vi "sample method.vi"(6 "Sample Commands":T2=enum."Index", 8 "error in (no error)":errorcluster, 9 "total run time":dbl[unit] format="%<%H:%M:%S%0u>t", 10 "current time":dbl[unit] format="%<%H:%M:%S>t", 11 "Ref cluster":T1) -> (0 "error out":errorcluster)   [LabVIEW 2012]
uses:
  Sample commands.ctl
  sample references.ctl
panel:
  in  "right white space":dbl=10.0
  in  "left white space":dbl=40.0
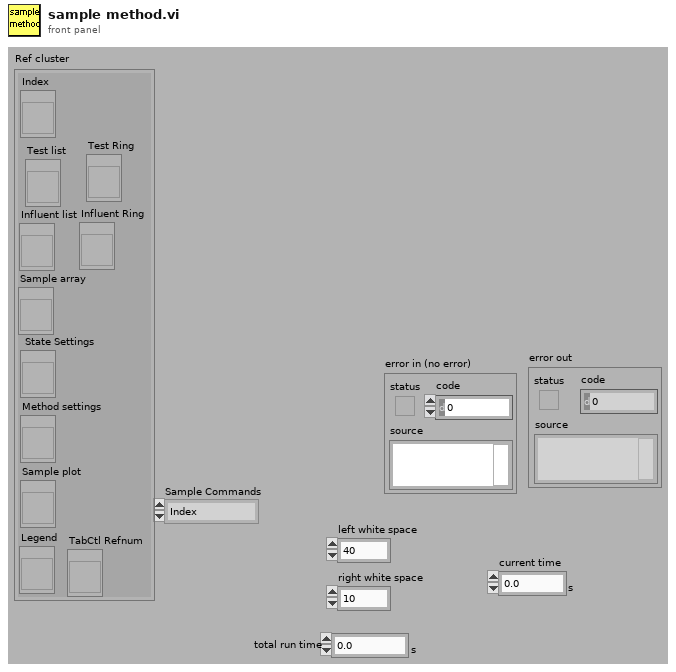
[diagram p1: front panel]
types:
  T1 = typedef "sample references.ctl" = cluster{"Index":refnum<vi>, "Test list":refnum<vi>, "Influent list":refnum<vi>, " State Settings":refnum<vi>, "Method settings":refnum<vi>, "Sample plot":refnum<vi>, "Legend":refnum<vi>, "Test Ring":refnum<vi>, "Influent Ring":refnum<vi>, "TabCtl Refnum":refnum<vi>, "Sample array":refnum<vi>}
  T2 = typedef "Sample commands.ctl" = enum16{"Configure", "Update times", "Index", "Update rings", "Plot current time"}
  T3 = cluster{"Width":u16, "Style":enum32{"Solid", "Dash", "Dot", "DashDot", "DashDotDot"}}
  T4 = typedef "Samples.ctl" = cluster{"start time":dbl[unit], "end time":dbl[unit], "state":string, "cycle":u16, "state":u16}[]
  T5 = cluster{"start time":dbl[unit], "end time":dbl[unit], "t/theta":dbl, "Test list":u16, "Influent list":u16, "Sample volume":dbl[unit], "Too close to previous sample":bool}[]
  T6 = typedef "LVBoundsTypeDef.ctl" = cluster{"Width":u32, "Height":u32}
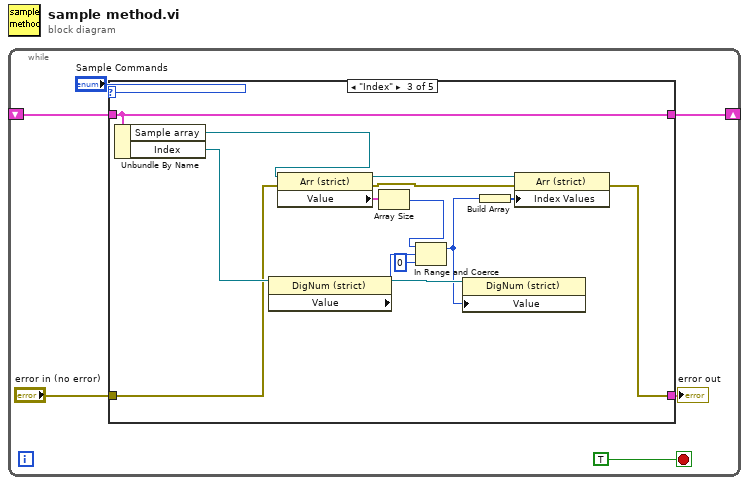
[diagram p0: block diagram]
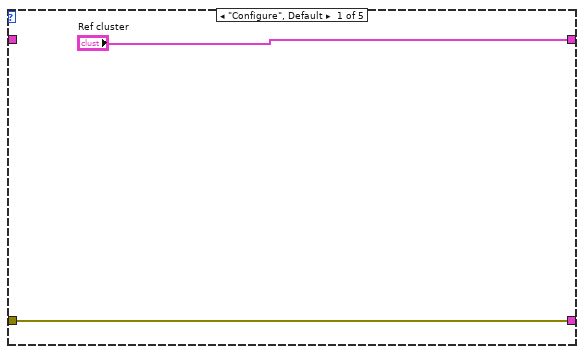
[diagram p2: hidden frame]
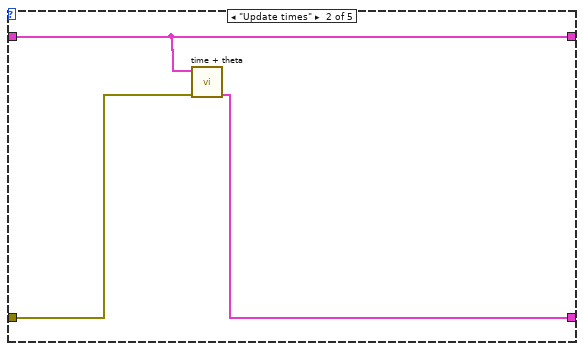
[diagram p3: hidden frame]
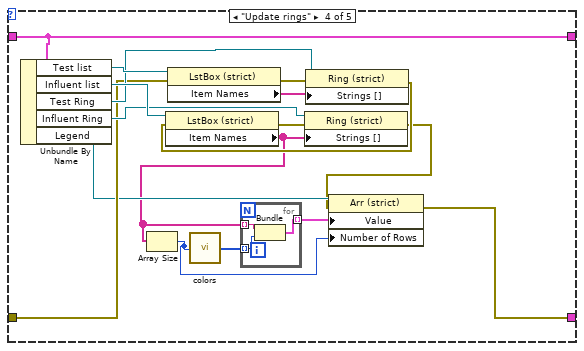
[diagram p4: hidden frame]
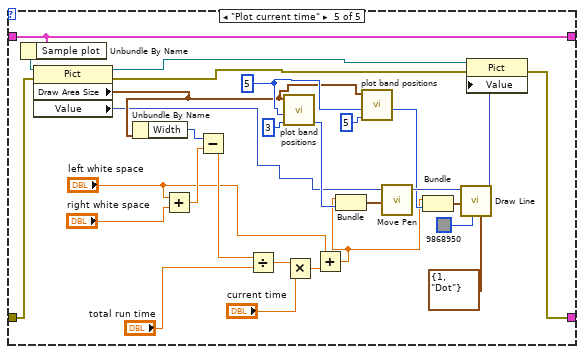
[diagram p5: hidden frame]
diagram:
  n1 = while {
    shift-right: [w4] -> _
    shift-left: _ -> [w3]
    stop <- TRUE stop-if-true
    n2 = case shown="\"Index\"" "Sample Commands" {
      tunnel: ["Ref cluster" w11 w15 w42 w54] -> w4
      tunnel: w3 -> [_ w11 w15 w42 w54]
      tunnel: "error in (no error)" -> [w8 w10 w14 w37 w48]
      tunnel: [w8 w9 w12 w27 w47] -> w1
      frame "Configure", Default {
      }
      frame "Update times" {
        n3 = call "time + theta.vi"("Sample start times"=w10, "Method settings"=w11) -> ("Samples"=w9:T4)  [unwired: 7 in, 2 out]
      }
      frame "Index" {
        n4 = Unbundle By Name(w15) -> ("Sample array"=w17:refnum<vi>, "Index"=w16:refnum<vi>)
        n5 = property class="DigNum (strict)"(reference=w16) -> (reference out=w20:refnum<vi>, "Value"=w21:i32)  [unwired: 1 in, 1 out]
        n6 = property class="Arr (strict)"(reference=w17, error in=w14) -> (reference out=w24:refnum<vi>, error out=w13:errorcluster, "Value"=w23:T5)
        n7 = Array Size(array=w23) -> (size(s)=w18:i32)
        n8 = In Range and Coerce(upper limit=w18, x=w21, lower limit=0) -> (coerced(x)=w19:i32)  [unwired: 1 out]
        n9 = property class="DigNum (strict)"(reference=w20, "Value"=w19) -> ()  [unwired: 1 in, 2 out]
        n10 = Build Array(w19) -> (w25:i32[])
        n11 = property class="Arr (strict)"(reference=w24, error in=w13, "Index Values"=w25) -> (error out=w12:errorcluster)  [unwired: 1 out]
      }
      frame "Update rings" {
        n12 = Unbundle By Name(w42) -> ("Test list"=w41:refnum<vi>, "Influent list"=w40:refnum<vi>, "Test Ring"=w39:refnum<vi>, "Influent Ring"=w38:refnum<vi>, "Legend"=w31:refnum<vi>)
        n13 = property class="LstBox (strict)"(reference=w41, error in=w37) -> (error out=w36:errorcluster, "Item Names"=w33:string[])  [unwired: 1 out]
        n14 = property class="Ring (strict)"(reference=w39, error in=w36, "Strings []"=w33) -> (error out=w35:errorcluster)  [unwired: 1 out]
        n15 = property class="LstBox (strict)"(reference=w40, error in=w35) -> (error out=w34:errorcluster, "Item Names"=w26:string[])  [unwired: 1 out]
        n16 = Array Size(array=w26) -> (size(s)=w30:i32)
        n17 = call "colors.vi"("colors needed"=w30) -> ("colors"=w32:u32[])
        n18 = for {
          tunnel: w26 -> [w45] mode=indexing
          tunnel: w32 -> [w44] mode=indexing
          tunnel: [w43] -> w29 mode=indexing
          n19 = Bundle(w45, "Color Box"=w44) -> (w43:cluster{string, "Color Box":u32})  [unwired: 1 in]
        }
        n20 = property class="Ring (strict)"(reference=w38, error in=w34, "Strings []"=w26) -> (error out=w28:errorcluster)  [unwired: 1 out]
        n21 = property class="Arr (strict)"(reference=w31, error in=w28, "Value"=w29, "Number of Rows"=w30) -> (error out=w27:errorcluster)  [unwired: 1 out]
      }
      frame "Plot current time" {
        w62 = i16 5 ("total bands")
        n22 = Unbundle By Name(w54) -> ("Sample plot"=w53:refnum<vi>)
        n23 = property class="Pict"(reference=w53, error in=w48) -> (reference out=w50:refnum<vi>, error out=w49:errorcluster, "Draw Area Size"=w52:T6, "Value"=w51:picture)
        n24 = Unbundle By Name(w52) -> ("Width"=w68:u32)
        n25 = Add(x="left white space", y="right white space") -> (x+y=w67:dbl)
        n26 = Subtract(x=w68, y=w67) -> (x-y=w61:dbl)
        n27 = Divide(x=w61, y="total run time") -> (x/y=w59:dbl[unit])
        n28 = call "plot band positions.vi"("band"=i16 3, "total bands"=w62, "Draw Area Size"=w52) -> ("bottom"=w64:u32)  [unwired: 2 in, 2 out]
        n29 = Multiply(x=w59, y="current time") -> (x*y=w57:dbl)
        n30 = Add(x="left white space", y=w57) -> (x+y=w55:dbl)
        n31 = Bundle(w55, "bottom"=w64) -> (w73:cluster{dbl, "bottom":u32})  [unwired: 1 in]
        n32 = call "plot band positions.vi"("band"=i16 5, "total bands"=w62, "Draw Area Size"=w52) -> ("top"=w63:u32)  [unwired: 2 in, 2 out]
        n33 = call <vilib>:"Move Pen.vi"("new position"=w73, "picture"=w51) -> ("new picture"=w74:picture)  [unwired: 3 in]
        n34 = Bundle(w55, "top"=w63) -> (w72:cluster{dbl, "top":u32})  [unwired: 1 in]
        n35 = call <vilib>:"Draw Line.vi"("picture"=w74, "end point"=w72, "color(black)"=u32 9868950, "pen"=T3 {"Width"=1, "Style"=enum."Dot"}) -> ("new picture"=w46:picture)  [unwired: 5 in]
        n36 = property class="Pict"(reference=w50, error in=w49, "Value"=w46) -> (error out=w47:errorcluster)  [unwired: 1 out]
      }
    }
    "error out" <- w1
  }
